vi "Pre Launch Init.vi"(11 "Accelerometer in":refnum<class "Accelerometer.lvclass">) -> (0 "error out":errorcluster, 3 "Accelerometer out":refnum<class "Accelerometer.lvclass">)   [LabVIEW 2020, in "Accelerometer.lvlib" / "Accelerometer.lvclass"]
doc: "Initializes the panel actor. Creates the Panel Helper.\n\n----\nPlease see the following web address for additional documentation and tutorial information:\nhttp://www.mooregoodideas.com/mgi-panel-manager/\n\nAuthor: Derek Trepanier\n\nCopyright (c) 2018, Moore Good Ideas, Inc.\n\nAll rights reserved.\n\nRedistribution and use in source and binary forms, with or without modification, are permitted provided that the following conditions are met:\n\n * Redistributions of source code must retain the above copyright notice, this list of conditions and the following disclaimer.\n * Redistributions in binary form must reproduce the above copyright notice, this list of conditions and the following disclaimer in the documentation and/or other materials provided with the distribution.\n * Neither the name of Moore Good Ideas, Inc. nor the names of its contributors may be used to endorse or promote products derived from this software without specific prior written permission.\n\nTHIS SOFTWARE IS PROVIDED BY THE COPYRIGHT HOLDERS AND CONTRIBUTORS \"AS IS\" AND ANY EXPRESS OR IMPLIED WARRANTIES, INCLUDING, BUT NOT LIMITED TO, THE IMPLIED WARRANTIES OF MERCHANTABILITY AND FITNESS FOR A PARTICULAR PURPOSE ARE DISCLAIMED. IN NO EVENT SHALL THE COPYRIGHT OWNER OR CONTRIBUTORS BE LIABLE FOR ANY DIRECT, INDIRECT, INCIDENTAL, SPECIAL, EXEMPLARY, OR CONSEQUENTIAL DAMAGES (INCLUDING, BUT NOT LIMITED TO, PROCUREMENT OF SUBSTITUTE GOODS OR SERVICES; LOSS OF USE, DATA, OR PROFITS; OR BUSINESS INTERRUPTION) HOWEVER CAUSED AND ON ANY THEORY OF LIABILITY, WHETHER IN CONTRACT, STRICT LIABILITY, OR TORT (INCLUDING NEGLIGENCE OR OTHERWISE) ARISING IN ANY WAY OUT OF THE USE OF THIS SOFTWARE, EVEN IF ADVISED OF THE POSSIBILITY OF SUCH DAMAGE."
uses:
  Accelerometer.lvclass
  Accel task df.ctl
  Accelerometer.lvclass/Accelerometer.ctl
  <vilib>/MGI/Panel Manager/Panel Actor/Panel Actor/Panel Actor.lvclass
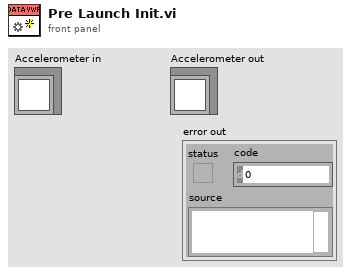
[diagram p1: front panel]
types:
  T1 = typedef "Accel task df.ctl" = enum16{"Idle", "Acquire", "Stop Helper Loop"}
  T2 = cluster{"X axis":dbl, "Y axis":dbl, "Z axis":dbl, "Total Mag":dbl}
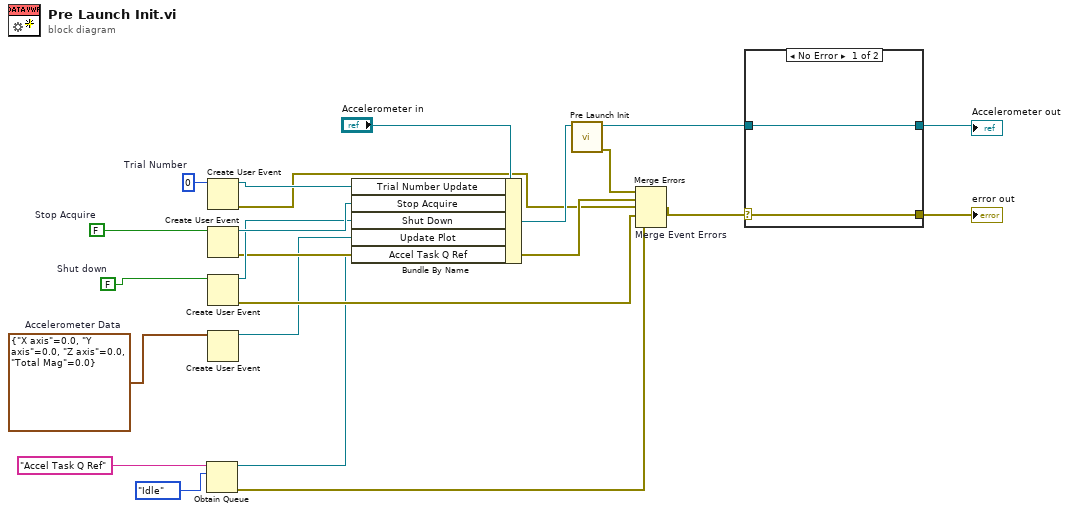
[diagram p0: block diagram]
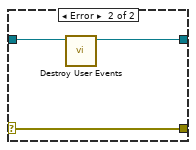
[diagram p2: hidden frame]
diagram:
  w5 = T2 {"X axis"=0.0, "Y axis"=0.0, "Z axis"=0.0, "Total Mag"=0.0}  # Accelerometer Data
  w15 = 0  # Trial Number
  w13 = FALSE  # Shut down
  w14 = FALSE  # Stop Acquire
  n1 = Obtain Queue(name (unnamed)="Accel Task Q Ref", element data type=Accel_task_df."Idle" ("Accel Enum")) -> (queue out=w2:refnum<queue>, error out=w1:errorcluster)  [unwired: 3 in, 1 out]
  n2 = Create User Event(user event datatype=w15) -> (user event=w12:refnum<user-event>, error out=w7:errorcluster)  [unwired: 1 in]
  n3 = Create User Event(user event datatype=w14) -> (user event=w11:refnum<user-event>, error out=w8:errorcluster)  [unwired: 1 in]
  n4 = Create User Event(user event datatype=w13) -> (user event=w10:refnum<user-event>, error out=w9:errorcluster)  [unwired: 1 in]
  n5 = Create User Event(user event datatype=w5) -> (user event=w6:refnum<user-event>)  [unwired: 1 in, 1 out]
  n6 = Bundle By Name(cluster="Accelerometer in", "Trial Number Update"=w12, "Stop Acquire"=w11, "Shut Down"=w10, "Update Plot"=w6, "Accel Task Q Ref"=w2) -> (w21:refnum<class "Accelerometer.lvclass">)
  n7 = call-parent "Pre Launch Init.vi"("Panel Actor in"=w21) -> ("error out"=w20:errorcluster, "Panel Actor out"=w19:refnum<class "Accelerometer.lvclass">)  [unwired: 9 in]
  n8 = Merge Errors "Merge Event Errors"(w20, w8, w7, w9, w1) -> (w18:errorcluster)
  n9 = case shown="No Error" w18 {
    selector: w18 -> [w24 w27]
    tunnel: w19 -> [w23 w26]
    tunnel: [w24 w27] -> w17
    tunnel: [w23 w25] -> w16
    frame No Error {
    }
    frame Error {
      n10 = call "Destroy User Events.vi"("Accelerometer in"=w26) -> ("Accelerometer out"=w25:refnum<class "Accelerometer.lvclass">)  [unwired: 10 in]
    }
  }
  "error out" <- w17
  "Accelerometer out" <- w16
